vi "Configure Frequency (Start Stop).vi"(8 "error in (no error)":errorcluster, 9 "Stop Frequency (2.65E+10 Hz)":dbl=26500000000.0, 10 "Start Frequency (1E+7 Hz)":dbl=10000000.0, 11 "VISA resource name":refnum<visa-resource-name>) -> (0 "error out":errorcluster, 3 "VISA resource name out":refnum<visa-resource-name>)   [LabVIEW 2018, in "Agilent MXA Series.lvlib"]
doc: "Configures the frequency range defining its start frequency and its stop frequency. If the start frequency is equal to the stop frequency, then the spectrum analyzer operates in the time-domain mode. Otherwise, the spectrum analyzer operates in frequency-domain mode."
uses:
  Agilent MXA Series.lvlib
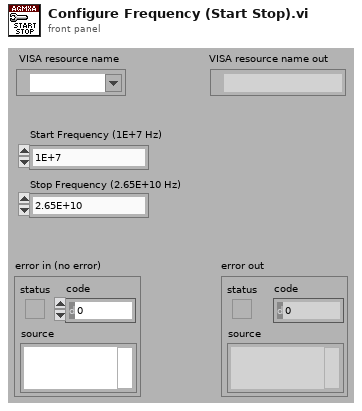
[diagram p1: front panel]
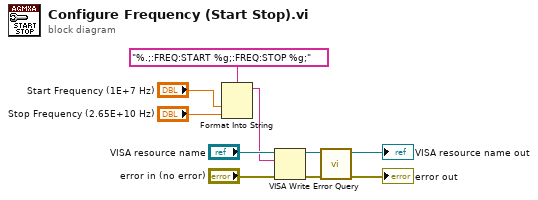
[diagram p0: block diagram]
diagram:
  n1 = Format Into String(format string="%.;:FREQ:START %g;:FREQ:STOP %g;", "Start Frequency (1E+7 Hz)", "Stop Frequency (2.65E+10 Hz)") -> (resulting string=w8:string)  [unwired: 2 in, 1 out]
  n2 = VISA Write(VISA resource name="VISA resource name", write buffer=w8, error in (no error)="error in (no error)") -> (VISA resource name out=w4:refnum<visa-resource-name>, error out=w2:errorcluster)  [unwired: 1 out]
  n3 = call "Error Query.vi"("error in (no error)"=w2, "VISA resource name"=w4) -> ("error out"=→"error out":errorcluster, "VISA resource name out"=→"VISA resource name out":refnum<visa-resource-name>)  [unwired: 6 in, 2 out]
